vi "RGB to HSV.vi"(8 "error in (no error)":errorcluster, 9 "Blue":u8, 10 "Green":u8, 11 "Red":u8) -> (0 "error out":errorcluster, 1 "Value(%)":dbl format="%#_13g", 2 "Saturation(%)":dbl format="%#_13g", 3 "Hue(°)":dbl format="%#_13g")   [LabVIEW 2018, in "Colour Lab.lvlib"]
uses:
  Colour Lab.lvlib
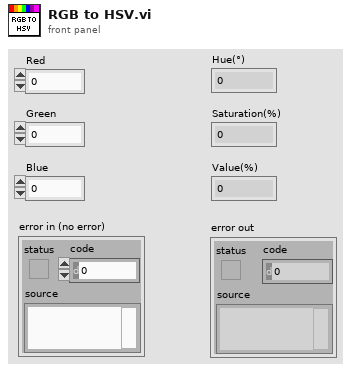
[diagram p1: front panel]
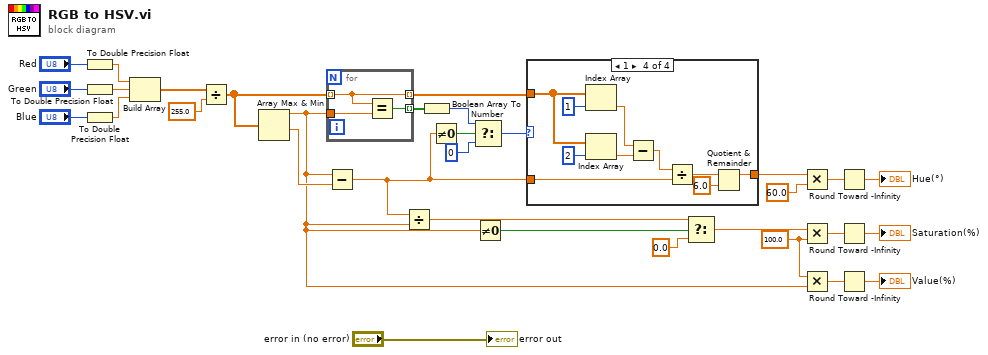
[diagram p0: block diagram]
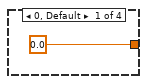
[diagram p2: hidden frame]
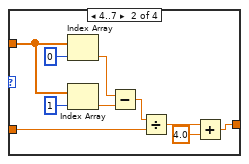
[diagram p3: hidden frame]
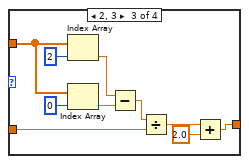
[diagram p4: hidden frame]
diagram:
  w18 = 100.0 ("x")
  n1 = To Double Precision Float(number="Red") -> (double precision float=w29:dbl)
  n2 = To Double Precision Float(number="Green") -> (double precision float=w28:dbl)
  n3 = To Double Precision Float(number="Blue") -> (double precision float=w27:dbl)
  n4 = Build Array(w29, w28, w27) -> (w26:dbl[])
  n5 = Divide(x=w26, y=255.0) -> (x/y=w14:dbl[])
  n6 = Array Max & Min(array=w14) -> (max value=w3:dbl, min value=w24:dbl)  [unwired: 2 out]
  n7 = for {
    tunnel: w3 -> [w35]
    tunnel: [w34] -> w15 mode=indexing
    tunnel: w14 -> [w33] mode=indexing
    tunnel: [w33] -> w13 mode=indexing
    n8 = Equal?(x=w33, y=w35) -> (x = y?=w34:bool)
  }
  n9 = Subtract(x=w3, y=w24) -> (x-y=w11:dbl)
  n10 = Divide(x=w11, y=w3) -> (x/y=w22:dbl)
  n11 = Boolean Array To Number(Boolean array=w15) -> (number=w9:u32)
  n12 = Not Equal To 0?(x=w11) -> (x != 0?=w10:bool)
  n13 = Select(t=w9, s=w10, f=u32 0) -> (s? t:f=w8:u32)
  n14 = Not Equal To 0?(x=w3) -> (x != 0?=w2:bool)
  n15 = case shown="1" w8 {
    tunnel: w13 -> [_ w39 w49 w62]
    tunnel: [0.0 ("x") w37 w47 w57] -> w12
    tunnel: w11 -> [_ w38 w48 w65]
    frame 0, Default {
    }
    frame 4..7 {
      n16 = Index Array(array=w39, index=0) -> (element=w42:dbl)
      n17 = Index Array(array=w39, index=1) -> (element=w41:dbl)
      n18 = Subtract(x=w42, y=w41) -> (x-y=w40:dbl)
      n19 = Divide(x=w40, y=w38) -> (x/y=w45:dbl)
      n20 = Add(x=w45, y=4.0) -> (x+y=w37:dbl)
    }
    frame 2, 3 {
      n21 = Index Array(array=w49, index=2) -> (element=w52:dbl)
      n22 = Index Array(array=w49, index=0) -> (element=w51:dbl)
      n23 = Subtract(x=w52, y=w51) -> (x-y=w50:dbl)
      n24 = Divide(x=w50, y=w48) -> (x/y=w55:dbl)
      n25 = Add(x=w55, y=2.0) -> (x+y=w47:dbl)
    }
    frame 1 {
      n26 = Index Array(array=w62, index=1) -> (element=w60:dbl)
      n27 = Index Array(array=w62, index=2) -> (element=w59:dbl)
      n28 = Subtract(x=w60, y=w59) -> (x-y=w58:dbl)
      n29 = Divide(x=w58, y=w65) -> (x/y=w64:dbl)
      n30 = Quotient & Remainder(x=w64, y=6.0) -> (x-y*floor(x/y)=w57:dbl)  [unwired: 1 out]
    }
  }
  n31 = Select(t=w22, s=w2, f=0.0 ("x")) -> (s? t:f=w20:dbl)
  n32 = Multiply(x=w12, y=60.0) -> (x*y=w17:dbl)
  n33 = Multiply(x=w20, y=w18) -> (x*y=w21:dbl)
  n34 = Multiply(x=w18, y=w3) -> (x*y=w19:dbl)
  n35 = Round Toward -Infinity(1:w17) -> (0:→"Hue(°)":dbl)
  n36 = Round Toward -Infinity(1:w21) -> (0:→"Saturation(%)":dbl)
  n37 = Round Toward -Infinity(1:w19) -> (0:→"Value(%)":dbl)
  "error out" <- "error in (no error)"
